vi "1_Placeholder - OptimizingWorkingDistance (SubVI).vi"(8 "error in (no error)":errorcluster, 10 "Image Array in":T1[](array[typedef]), 11 "Captured positions":dbl[][](array[numeric])) -> (0 "error out":errorcluster, 2 "Image Array out":T1[](array[typedef]), 3 "Optimized working distance":dbl)   [LabVIEW 2016]
uses:
  <vilib>/vision/Image Controls.llb/IMAQ Image.ctl
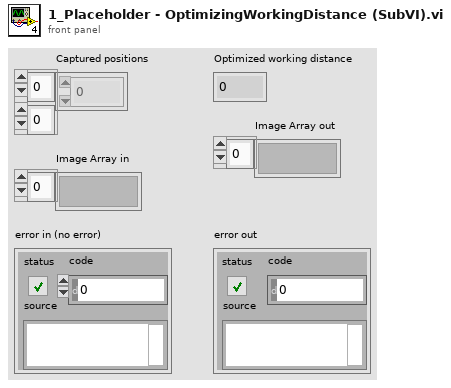
[diagram p1: front panel]
types:
  T1 = typedef "IMAQ Image.ctl" = refnum<image>
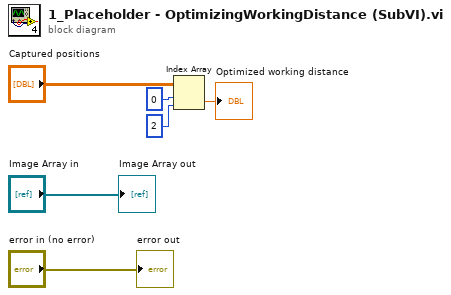
[diagram p0: block diagram]
diagram:
  n1 = Index Array(array="Captured positions", index (row)=0, index (col)=2 ("disabled index (col)")) -> (element=→"Optimized working distance":dbl)
  "Image Array out" <- "Image Array in"
  "error out" <- "error in (no error)"
